vi "Clear Errors.vi"(4 "error in (no error)":errorcluster caption="错误输入（无错误）", 7 "specific error code to clear (0: all)":i32 caption="清除指定错误代码（0：全部代码）") -> (0 "error out":errorcluster caption="错误输出", 3 "specific error cleared?":bool caption="指定错误已清除？")   [LabVIEW 2018]
doc: "将错误<B>状态</B>重置为无错误，<B>代码</B>重置为0，<B>源</B>重置为空字符串。 使用该VI来忽略一个错误。 默认情况下，VI忽略全部错误。 如需忽略特定错误，连线错误代码值至<B>清空特定错误代码</B>。"
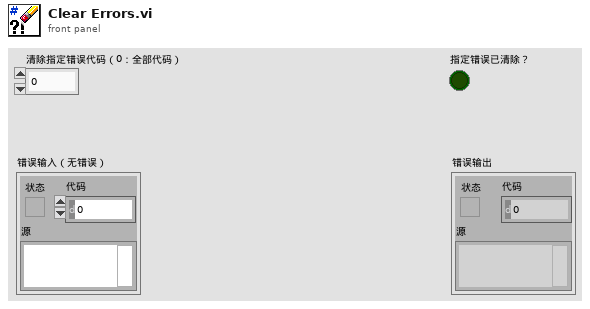
[diagram p1: front panel]
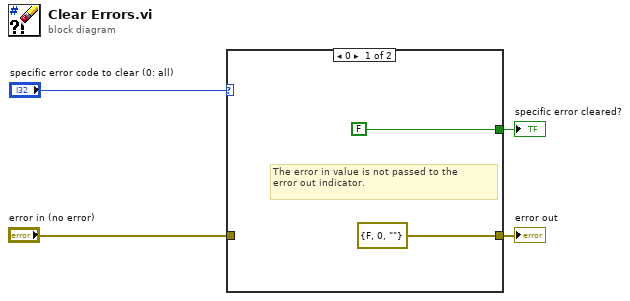
[diagram p0: block diagram]
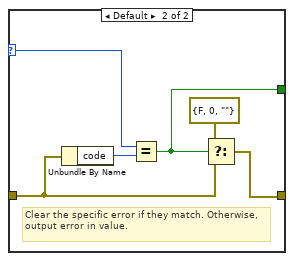
[diagram p2: hidden frame]
diagram:
  n1 = case shown="0" "specific error code to clear (0: all)" {
    selector: "specific error code to clear (0: all)" -> [_ w11]
    tunnel: "error in (no error)" -> [_ w10]
    tunnel: [errorcluster {"status"=FALSE, "code"=0, "source"=""} ("error constant") w7] -> w2
    tunnel: [FALSE w8] -> w1
    frame 0 {
      # "The error in value is not passed to the\nerror out indicator."
    }
    frame Default {
      # "Clear the specific error if they match. Otherwise, output error in value."
      n2 = Unbundle By Name(w10) -> ("code"=w12:i32)
      n3 = Equal?(x=w11, y=w12) -> (x = y?=w8:bool)
      n4 = Select(t=errorcluster {"status"=FALSE, "code"=0, "source"=""} ("error constant"), s=w8, f=w10) -> (s? t:f=w7:errorcluster)
    }
  }
  "error out" <- w2
  "specific error cleared?" <- w1
